vi "main1.0.vi"() -> ()   [LabVIEW 2018]
uses:
  <vilib>/Analysis/baseanly.llb/Mean (DBL).vi
  <vilib>/Instr/_visa.llb/VISA Configure Serial Port (Instr).vi
  <vilib>/Analysis/NI_AALBase.lvlib
panel:
  out "示波器采集":bool
  out "单片机控制":bool
  in  "示波器通信端口":refnum<visa-resource-name>="USB0::0x0957::0x1754::MY48260178::INSTR"
  out "二支":bool
  out "一支":bool
  in  "布尔":bool caption="双路选择"
  out "正峰":dbl
  out "反峰":dbl
  out "峰峰值":dbl
  out "Waveform Data":waveform(dbl)(graph)
  out "字符串":string
  out "2-7 2":bool
  out "2-6 2":bool
  out "2-5 2":bool
  out "2-4 2":bool
  out "2-3 2":bool
  out "2-2 2":bool
  out "2-1 2":bool
  out "1-7 2":bool
  out "1-6 2":bool
  out "1-5 2":bool
  out "1-4 2":bool
  out "1-3 2":bool
  out "1-2 2":bool
  out "1-1 2":bool
  out "读取缓冲区":string
  in  "单片机COM":refnum<visa-resource-name>
  in  "1-7":bool
  in  "2-7":bool
  in  "2-6":bool
  in  "2-5":bool
  in  "2-4":bool
  in  "2-3":bool
  in  "2-2":bool
  in  "2-1":bool
  in  "1-1":bool
  in  "1-2":bool
  in  "1-3":bool
  in  "1-4":bool
  in  "1-5":bool
  in  "1-6":bool
  out "文件存储":bool
  in  "数据存储位置（文件名称:触发采集时间）":path
  in  "触发采集":bool
  # "单路"
  # "双路"
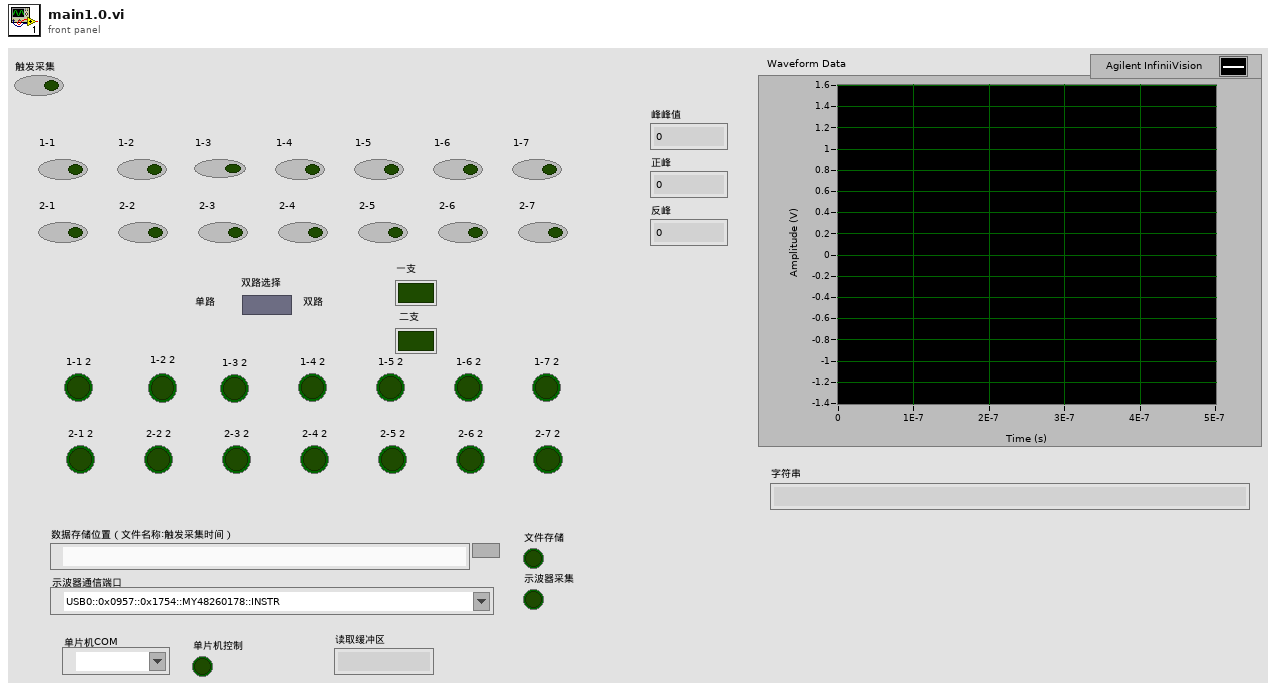
[diagram p1: front panel]
types:
  T1 = enum16{"open", "replace", "create", "open or create", "replace or create", "replace or create with confirmation"}
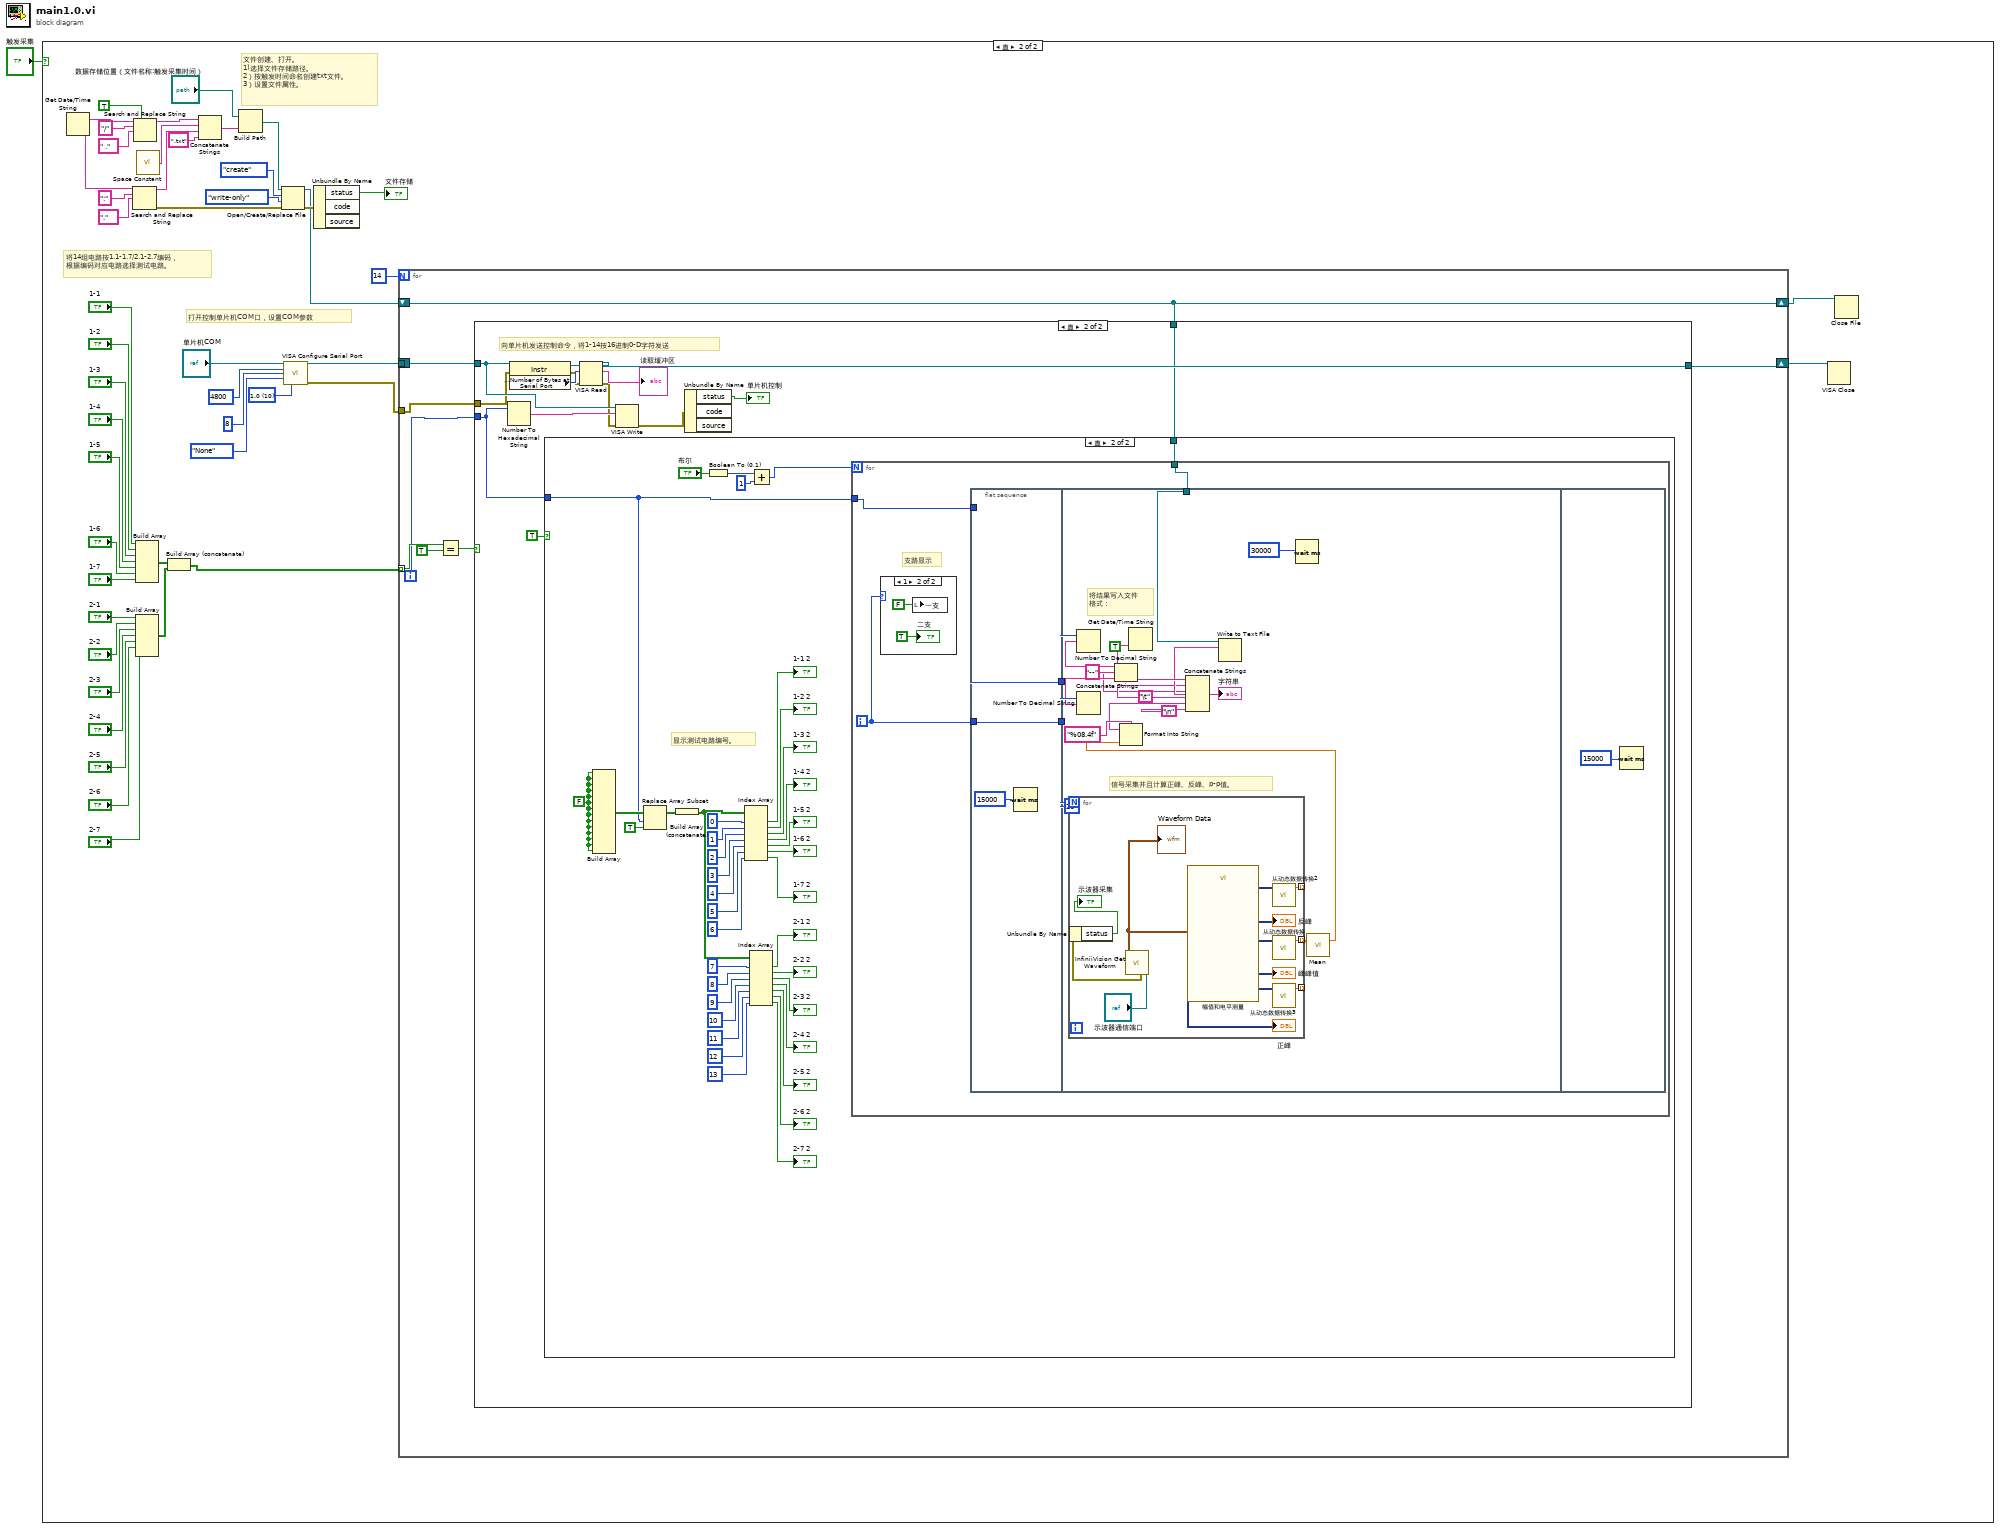
[diagram p0: block diagram]
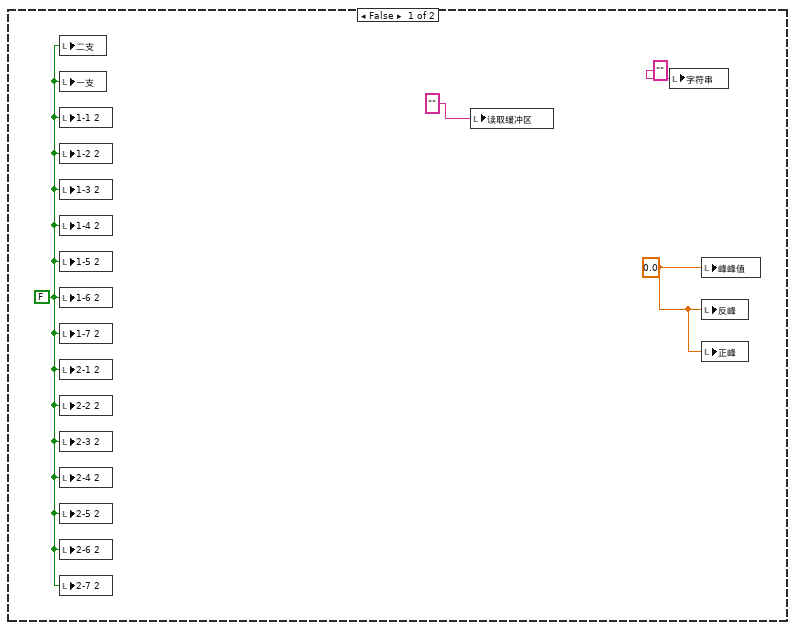
[diagram p2: hidden frame]
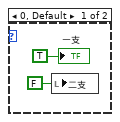
[diagram p5: hidden frame]
diagram:
  n1 = case shown="真" "触发采集" {
    frame False {
      w3 = 0.0 ("峰峰值")
      w2 = FALSE
      n2 = local write "二支"(w2) -> ()
      n3 = local write "一支"(w2) -> ()
      n4 = local write "1-1 2"(w2) -> ()
      n5 = local write "1-2 2"(w2) -> ()
      n6 = local write "1-3 2"(w2) -> ()
      n7 = local write "1-4 2"(w2) -> ()
      n8 = local write "1-5 2"(w2) -> ()
      n9 = local write "1-6 2"(w2) -> ()
      n10 = local write "1-7 2"(w2) -> ()
      n11 = local write "2-1 2"(w2) -> ()
      n12 = local write "2-2 2"(w2) -> ()
      n13 = local write "2-3 2"(w2) -> ()
      n14 = local write "2-4 2"(w2) -> ()
      n15 = local write "2-5 2"(w2) -> ()
      n16 = local write "2-6 2"(w2) -> ()
      n17 = local write "2-7 2"(w2) -> ()
      n18 = local write "读取缓冲区"("" ("读取缓冲区")) -> ()
      n19 = local write "字符串"("" ("字符串")) -> ()
      n20 = local write "峰峰值"(w3) -> ()
      n21 = local write "反峰"(w3) -> ()
      n22 = local write "正峰"(w3) -> ()
    }
    frame True {
      w15 = u16 10 items=["1.0"=10, "1.5"=15, "2.0"=20] ("stop bits (10: 1 bit)")
      # "打开控制单片机COM口，设置COM参数"
      # "将14组电路按1.1-1.7/2.1-2.7编码，\n根据编码对应电路选择测试电路。"
      # "文件创建、打开。\n1)选择文件存储路径。\n2）按触发时间命名创建txt文件。\n3）设置文件属性。"
      n23 = Get Date/Time String() -> (date string=w48:string, time string=w50:string)  [unwired: 3 in]
      n24 = Search and Replace String(input string=w50, search string=":", replace string=".") -> (result string=w47:string, error out=w43:errorcluster)  [unwired: 5 in, 2 out]
      n25 = Search and Replace String(replace all?=TRUE, input string=w48, search string="/", replace string=" .") -> (result string=w44:string)  [unwired: 4 in, 3 out]
      n26 = Build Array("1-1", "1-2", "1-3", "1-4", "1-5", "1-6", "1-7") -> (w20:bool[])
      n27 = Build Array("2-1", "2-2", "2-3", "2-4", "2-5", "2-6", "2-7") -> (w19:bool[])
      n28 = call <vilib>:"Space Constant.vi"() -> ("String"=w49:string)
      n29 = Build Array (concatenate)(w20, w19) -> (w11:bool[])
      n30 = Concatenate Strings(w44, w49, w47, ".txt") -> (w52:string)
      n31 = Build Path(base path="数据存储位置（文件名称:触发采集时间）", name or relative path=w52) -> (appended path=w51:path)
      n32 = Open/Create/Replace File(file path (use dialog)=w51, error in=w43, operation (0:open)=T1."create", access (0:read/write)=enum16{"read/write", "read-only", "write-only"}."write-only") -> (refnum out=w10:refnum<file>, error out=w45:errorcluster)  [unwired: 3 out]
      n33 = call-poly "VISA Configure Serial Port"("VISA resource name"="单片机COM", "baud rate (9600)"=4800, "data bits (8)"=u16 8, "parity (0:none)"=enum16{"None", "Odd", "Even", "Mark", "Space"}."None", "stop bits (10: 1 bit)"=w15) -> ("VISA resource name out"=w12:refnum<visa-resource-name>, "error out"=w7:errorcluster)  [unwired: 9 in]
      n34 = Unbundle By Name(w45) -> ("status"=→"文件存储":bool)  [unwired: 2 out]
      n35 = for {
        N: 14 -> [_]
        tunnel: w12 -> [w56]
        tunnel: w11 -> [w60] mode=indexing
        shift-right: [w54] -> w9
        shift-left: w10 -> [w54]
        shift-right: [w55] -> w8
        shift-left: _ -> [_]
        tunnel: w7 -> [w53]
        i -> [w57]
        n36 = Equal?(x=w60, y=TRUE) -> (x = y?=w58:bool)
        n37 = case shown="真" w58 {
          tunnel: w57 -> [_ w69]
          tunnel: w56 -> [w61 w72]
          tunnel: [w61 w71] -> w55
          tunnel: w54 -> [_ w70]
          tunnel: w53 -> [_ w66]
          frame False {
          }
          frame True {
            # "向单片机发送控制命令，将1-14按16进制0-D字符发送"
            n38 = Number To Hexadecimal String(2:w69) -> (0:w75:string)  [unwired: 1 in]
            n39 = property class="Instr"(reference=w72, error in=w66) -> (reference out=w74:refnum<visa-resource-name>, error out=w67:errorcluster, "Serial Settings:Number of Bytes at Serial Port"=w73:u32)
            n40 = case shown="真" TRUE {
              tunnel: w70 -> [_ w82]
              tunnel: w69 -> [_ w80]
              frame False {
              }
              frame True {
                w114 = FALSE
                # "显示测试电路编号。"
                n41 = Build Array(w114, w114, w114, w114, w114, w114, w114, w114, w114, w114, w114, w114, w114, w114) -> (w81:bool[])
                n42 = Replace Array Subset(array=w81, new element=TRUE, index=w80) -> (w83:bool[])
                n43 = Build Array (concatenate)(w83) -> (w98:bool[])
                n44 = Boolean To (0,1)(Boolean="布尔") -> (0, 1=w78:i16)
                n45 = Index Array(array=w98, index #1=0, index #2=1, index #3=2, index #4=3, index #5=4, index #6=5, index #7=6) -> (element #1=→"1-1 2":bool, element #2=→"1-2 2":bool, element #3=→"1-3 2":bool, element #4=→"1-4 2":bool, element #5=→"1-5 2":bool, element #6=→"1-6 2":bool, element #7=→"1-7 2":bool)
                n46 = Add(x=w78, y=1) -> (x+y=w76:i32)
                n47 = Index Array(array=w98, index #1=7, index #2=8, index #3=9, index #4=10, index #5=11, index #6=12, index #7=13) -> (element #1=→"2-1 2":bool, element #2=→"2-2 2":bool, element #3=→"2-3 2":bool, element #4=→"2-4 2":bool, element #5=→"2-5 2":bool, element #6=→"2-6 2":bool, element #7=→"2-7 2":bool)
                n48 = for {
                  N: w76 -> [_]
                  tunnel: w82 -> [w118]
                  tunnel: w80 -> [w117]
                  i -> [w115]
                  # "支路显示"
                  n49 = case shown="1" w115 {
                    frame 0, Default {
                      n50 = local write "二支"(FALSE) -> ()
                      "一支" <- TRUE
                    }
                    frame 1 {
                      n51 = local write "一支"(FALSE) -> ()
                      "二支" <- TRUE
                    }
                  }
                  n52 = flat-sequence {
                    tunnel: w117 -> [w125]
                    tunnel: [w125] -> w119
                    tunnel: w115 -> [w124]
                    tunnel: [w124] -> w116
                    tunnel: w118 -> [w137]
                    tunnel: w119 -> [w132]
                    tunnel: w116 -> [w131]
                    frame #0 {
                      n53 = Wait (ms)(milliseconds to wait=u32 15000 ("等待时间（毫秒）")) -> ()  [unwired: 1 out]
                    }
                    frame #1 {
                      w139 = "\t" ("Tab")
                      # "信号采集并且计算正峰、反峰、p-p值。"
                      # "将结果写入文件\n格式："
                      n54 = for {
                        N: 20 -> [_]
                        tunnel: [w152] -> w136 mode=indexing
                        tunnel: [w149] -> _ mode=indexing
                        tunnel: [w148] -> _ mode=indexing
                        n55 = call "InfiniiVision Get Waveform.vi"("VISA Resource Name"="示波器通信端口") -> ("error out"=w146:errorcluster, "Waveform Data"=w154:waveform(dbl))  [unwired: 9 in]
                        "Waveform Data" <- w154
                        n56 = Unbundle By Name(w146) -> ("status"=→"示波器采集":bool)
                        n57 = call "幅值和电平测量"("Signals"=w154) -> ("Negative Peak"=w151:dynamicdata, "Positive Peak"=w150:dynamicdata, "Peak to Peak"=w153:dynamicdata)  [unwired: 11 in, 1 out]
                        "峰峰值" <- w153
                        "反峰" <- w151
                        "正峰" <- w150
                        n58 = call "从动态数据转换2"("Dynamic Data Type"=w151) -> ("Scalar"=w148:dbl)  [unwired: 3 in]
                        n59 = call "从动态数据转换"("Dynamic Data Type"=w153) -> ("Scalar"=w152:dbl)  [unwired: 3 in]
                        n60 = call "从动态数据转换3"("Dynamic Data Type"=w150) -> ("Scalar"=w149:dbl)  [unwired: 3 in]
                      }
                      n61 = Number To Decimal String(number=w132) -> (decimal integer string=w130:string)  [unwired: 1 in]
                      n62 = Number To Decimal String(number=w131) -> (decimal integer string=w129:string)  [unwired: 1 in]
                      n63 = Concatenate Strings(w130, "--", w129) -> (w127:string)
                      n64 = Get Date/Time String(want seconds? (F)=TRUE) -> (time string=w142:string)  [unwired: 2 in, 1 out]
                      n65 = Wait (ms)(milliseconds to wait=u32 30000 ("等待时间（毫秒）")) -> ()  [unwired: 1 out]
                      n66 = call-poly <vilib>:"Mean.vi"("X"=w136) -> ("mean"=w133:dbl)  [unwired: 1 out]
                      n67 = Format Into String(format string="%08.4f" ("格式字符串"), w133) -> (resulting string=w134:string)  [unwired: 2 in, 1 out]
                      n68 = Concatenate Strings(w142, w139, w127, w139, w134, "\n") -> (w141:string)
                      "字符串" <- w141
                      n69 = Write to Text File(file (use dialog)=w137, text=w141) -> ()  [unwired: 2 in, 3 out]
                    }
                    frame #2 {
                      n70 = Wait (ms)(milliseconds to wait=u32 15000 ("等待时间（毫秒）")) -> ()  [unwired: 1 out]
                    }
                  }
                }
              }
            }
            n71 = VISA Read(VISA resource name=w74, byte count=w73, error in (no error)=w67) -> (VISA resource name out=w71:refnum<visa-resource-name>, read buffer=→"读取缓冲区":string, error out=w64:errorcluster)  [unwired: 1 out]
            n72 = VISA Write(VISA resource name=w72, write buffer=w75, error in (no error)=w64) -> (error out=w63:errorcluster)  [unwired: 2 out]
            n73 = Unbundle By Name(w63) -> ("status"=→"单片机控制":bool)  [unwired: 2 out]
          }
        }
      }
      n74 = VISA Close(VISA resource name=w8) -> ()  [unwired: 1 in, 1 out]
      n75 = Close File(refnum=w9) -> ()  [unwired: 1 in, 2 out]
    }
  }
